vi "DIM_Read Sourcers.SysLabels.vi"(8 "error in (no error)":errorcluster, 11 "UI_Actor in":refnum<class "UI_Actor.lvclass">) -> (0 "error out":errorcluster, 2 "DIM Sourcer.SysLabels":string[](array[string]), 3 "UI_Actor out":refnum<class "UI_Actor.lvclass">)   [LabVIEW 2020, in "UI_Actor.lvlib" / "UI_Actor.lvclass"]
uses:
  UI_Actor.lvclass
  UI_Actor.lvclass/UI_Actor.ctl
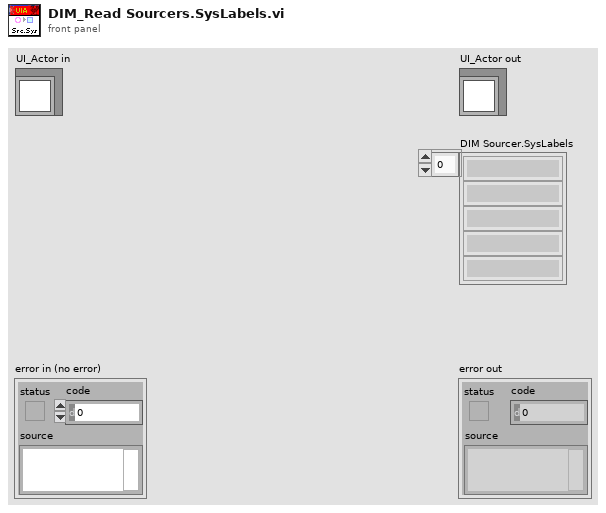
[diagram p1: front panel]
types:
  T1 = typedef "UI_Actor.lvlib/UI_Actor.lvclass/ctl_InternalMapItem.ctl" = cluster{"Config":refnum<class "Config.lvclass">, "LatestData":refnum<class "Data.lvclass">}
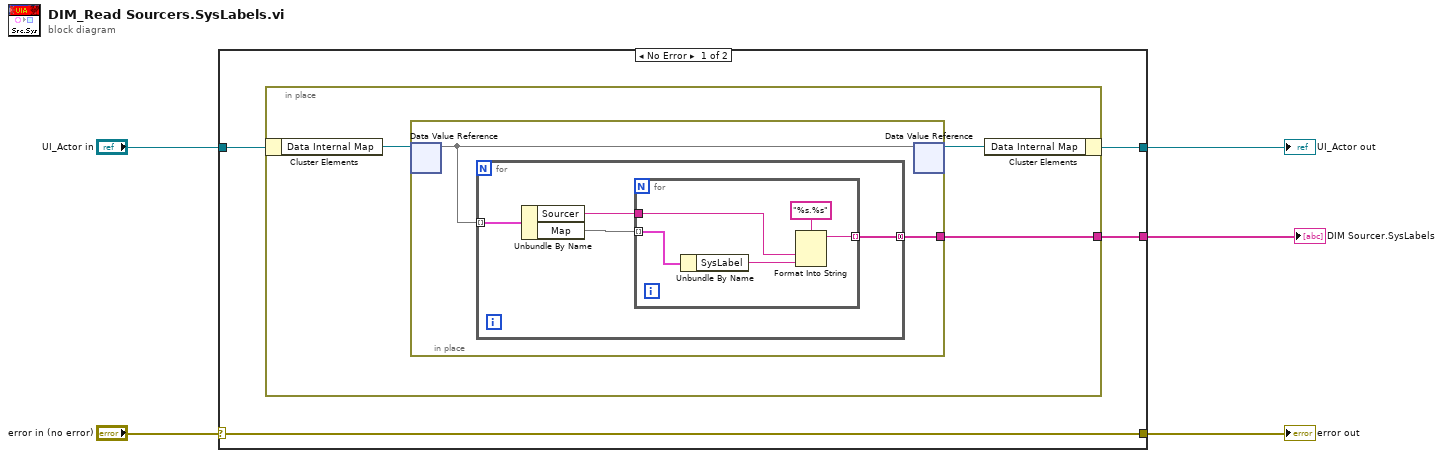
[diagram p0: block diagram]
diagram:
  n1 = case shown="No Error" "error in (no error)" {
    selector: "error in (no error)" -> [w9 w25]
    tunnel: [w9 w25] -> w4
    tunnel: [w7 w24] -> w2
    tunnel: "UI_Actor in" -> [w8 w24]
    tunnel: [w6 _] -> w1
    frame No Error {
      n2 = in-place {
        in-place-border: [w10] -> w6
        n3 = in-place-cluster #1(w8) -> ("Data Internal Map"=w12:refnum<data-value>)
        n4 = in-place {
          in-place-border: [w13] -> w10
          n5 = in-place-dvr #2(w12) -> (w14:map{string, map{string, T1}})  [unwired: 1 out]
          n6 = for {
            tunnel: w14 -> [w18] mode=indexing
            tunnel: [w15] -> w13 mode=concatenating
            n7 = Unbundle By Name(w18) -> ("Sourcer"=w16:string, "Map"=w17:map{string, T1})
            n8 = for {
              tunnel: w17 -> [w23] mode=indexing
              tunnel: w16 -> [w21]
              tunnel: [w19] -> w15 mode=indexing
              n9 = Unbundle By Name(w23) -> ("SysLabel"=w20:string)
              n10 = Format Into String(format string="%s.%s", w21, w20) -> (resulting string=w19:string)  [unwired: 2 in, 1 out]
            }
          }
          n11 = in-place-dvr #2(w14) -> (w11:refnum<data-value>)  [unwired: 1 out]
        }
        n12 = in-place-cluster #1("Data Internal Map"=w11) -> (w7:refnum<class "UI_Actor.lvclass">)
      }
    }
    frame Error {
    }
  }
  "error out" <- w4
  "UI_Actor out" <- w2
  "DIM Sourcer.SysLabels" <- w1
